vi "PROXY_REF_CHG_check_for_error.vi"(8 "PROXY_REF_CHG_sequence_state_in":T1, 11 "error_in":errorcluster) -> (0 "PROXY_REF_CHG_sequence_state_out":T1, 3 "error_out":errorcluster)   [LabVIEW 2020]
uses:
  PROXY_REF_CHG_sequence_state.ctl
  FGV/reference_change_connection/FGV_PROXY_REF_CHG_connection.ctl
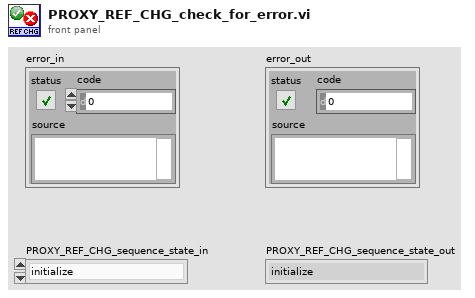
[diagram p1: front panel]
types:
  T1 = typedef "PROXY_REF_CHG_sequence_state.ctl" = enum16{"initialize", "wait_for_connection", "handle_message", "error", "stop"}
  T2 = typedef "FGV_PROXY_REF_CHG_connection.ctl" = enum16{"initialize", "set_listener_ID", "set_connection_ID", "get", "KILL CONNECTION", "killed?"}
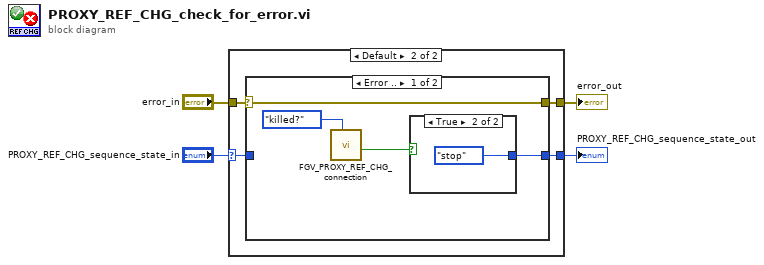
[diagram p0: block diagram]
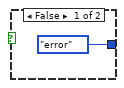
[diagram p3: hidden frame]
diagram:
  n1 = case shown="Default" "PROXY_REF_CHG_sequence_state_in" {
    selector: "PROXY_REF_CHG_sequence_state_in" -> [w5 w8]
    tunnel: [w6 w10] -> w4
    tunnel: [w5 w9] -> w3
    tunnel: "error_in" -> [w6 w7]
    frame "stop" {
    }
    frame Default {
      n2 = case shown="Error .." w7 {
        selector: w7 -> [w13 w17]
        tunnel: [w14 w18] -> w9
        tunnel: w8 -> [_ w18]
        tunnel: [w13 w17] -> w10
        frame Error {
          n3 = call "FGV_PROXY_REF_CHG_connection.vi"("options"=FGV_PROXY_REF_CHG_connection."killed?") -> ("killed?"=w12:bool)  [unwired: 7 in, 3 out]
          n4 = case shown="True" w12 {
            tunnel: [PROXY_REF_CHG_sequence_state."error" ("PLC_TCP_1_loop_states") PROXY_REF_CHG_sequence_state."stop" ("PLC_TCP_1_loop_states")] -> w14
            frame False {
            }
            frame True {
            }
          }
        }
        frame No Error {
        }
      }
    }
  }
  "error_out" <- w4
  "PROXY_REF_CHG_sequence_state_out" <- w3
